vi "Input.vi"() -> ()   [LabVIEW 2025]
uses:
  <userlib>/_NEVSTOP/Communicable State Machine(CSM)/Communicable State Machine.lvlib
panel:
  in  "stop":bool
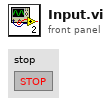
[diagram p1: front panel]
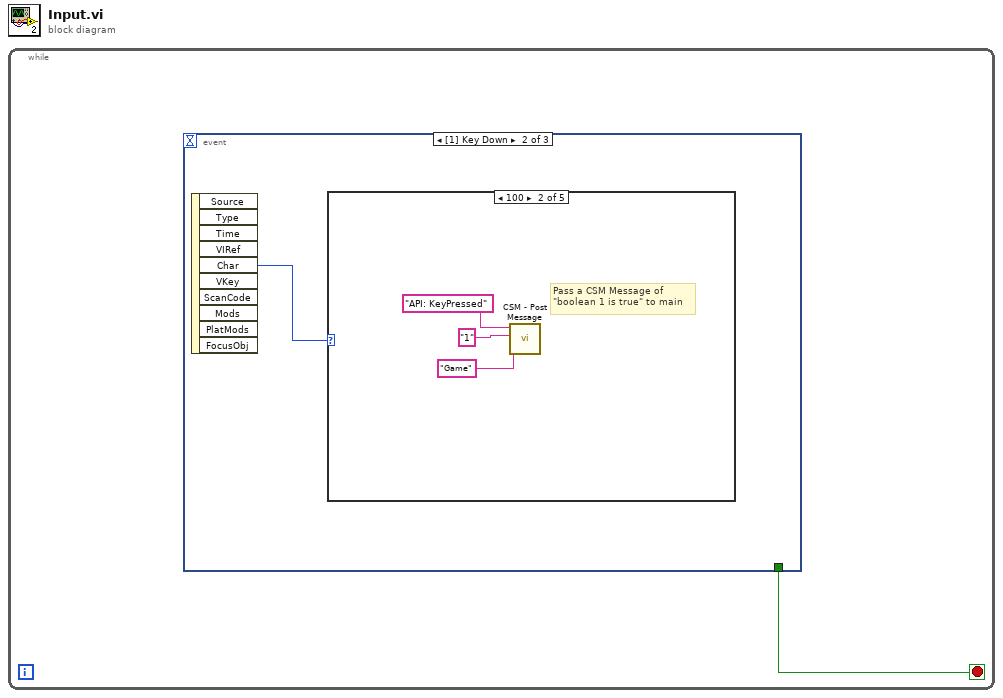
[diagram p0: block diagram]
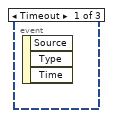
[diagram p2: hidden frame]
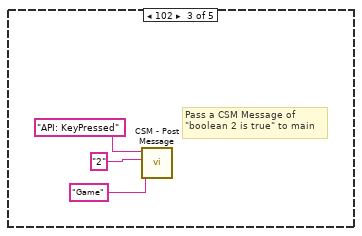
[diagram p4: hidden frame]
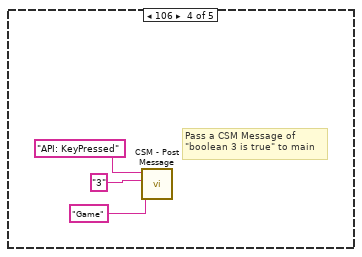
[diagram p5: hidden frame]
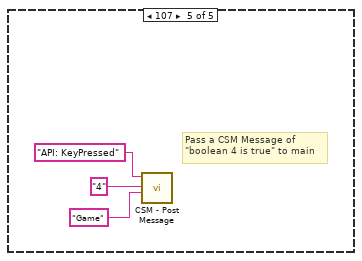
[diagram p6: hidden frame]
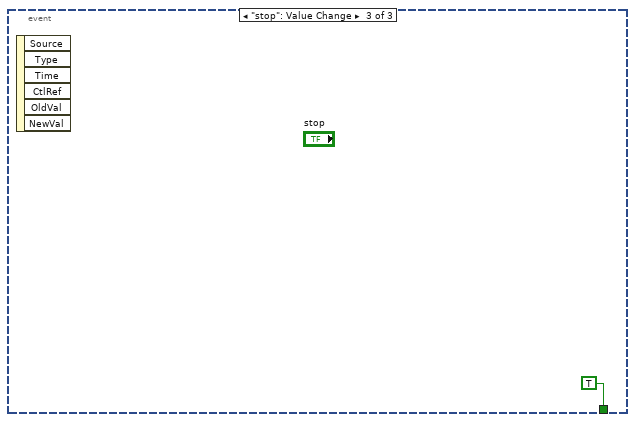
[diagram p7: hidden frame]
diagram:
  n1 = while {
    stop <- w1 stop-if-true
    n2 = event shown="[1] Key Down" {
      selector: _ -> [_ _ _]
      dyn-events: _ -> [_ _ _]
      timeout: _ -> [_ _ _]
      tunnel: [_ _ TRUE] -> w1
      event Timeout {
        n3 = event-data() -> ()  [unwired: 1 in, 3 out]
      }
      event Key Down {
        n4 = event-data() -> ("Char"=w2:i16)  [unwired: 1 in, 9 out]
        n5 = case shown="100" w2 {
          frame 0, Default {
          }
          frame 100 {
            # "Pass a CSM Message of \n\"boolean 1 is true\" to main"
            n6 = call <userlib>:"CSM - Post Message.vi"("Target Module"="Game", "Arguments (\"\")"="1" ("Arguments (\"\")"), "State"="API: KeyPressed") -> ()  [unwired: 8 in, 1 out]
          }
          frame 102 {
            # "Pass a CSM Message of \n\"boolean 2 is true\" to main"
            n7 = call <userlib>:"CSM - Post Message.vi"("Target Module"="Game", "Arguments (\"\")"="2" ("Arguments (\"\")"), "State"="API: KeyPressed") -> ()  [unwired: 8 in, 1 out]
          }
          frame 106 {
            # "Pass a CSM Message of \n\"boolean 3 is true\" to main"
            n8 = call <userlib>:"CSM - Post Message.vi"("Target Module"="Game", "Arguments (\"\")"="3" ("Arguments (\"\")"), "State"="API: KeyPressed") -> ()  [unwired: 8 in, 1 out]
          }
          frame 107 {
            # "Pass a CSM Message of \n\"boolean 4 is true\" to main"
            n9 = call <userlib>:"CSM - Post Message.vi"("Target Module"="Game", "Arguments (\"\")"="4" ("Arguments (\"\")"), "State"="API: KeyPressed") -> ()  [unwired: 8 in, 1 out]
          }
        }
      }
      event "stop": Value Change {
        n10 = event-data() -> ()  [unwired: 1 in, 6 out]
      }
    }
  }
